vi "To Pretty String (Object).vi"(6 "pretty print? (T)":bool=TRUE, 7 "enable LabVIEW extensions? (T)":bool=TRUE, 8 "error in (no error)":errorcluster, 10 "indent":i32, 11 "JSON Value in":refnum<class "JSON Value.lvclass">) -> (0 "error out":errorcluster, 3 "Pretty Print String":string)   [LabVIEW 2016, in "JSON Value.lvclass"]
doc: "Pretty prints the given JSON data in an easier to read format."
uses:
  JSON Value.lvclass
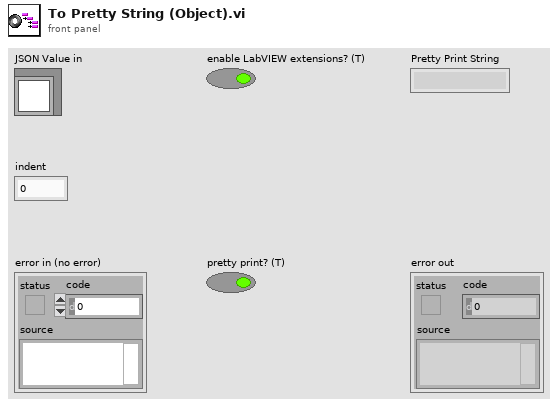
[diagram p1: front panel]
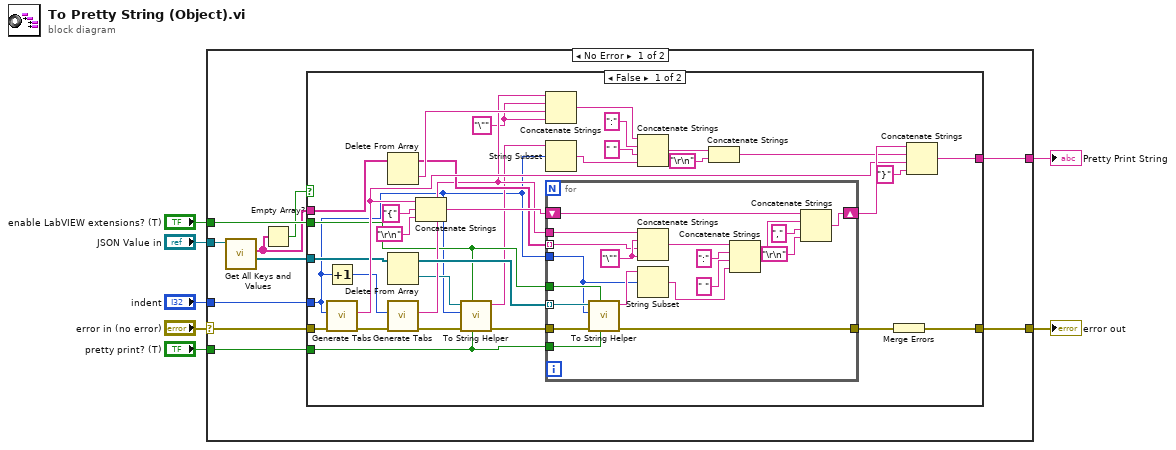
[diagram p0: block diagram]
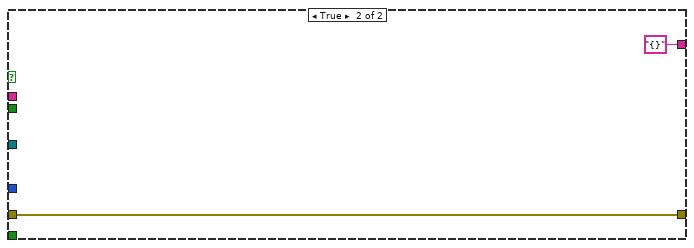
[diagram p2: hidden frame]
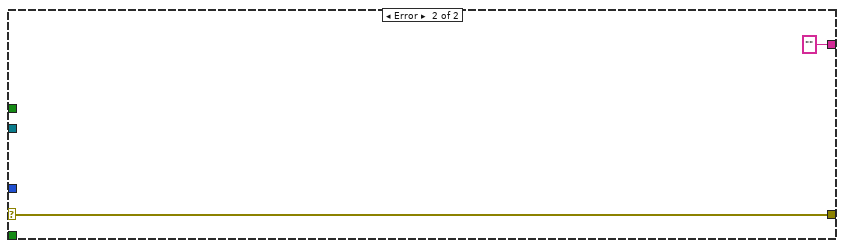
[diagram p3: hidden frame]
diagram:
  n1 = case shown="No Error" "error in (no error)" {
    selector: "error in (no error)" -> [w15 w72]
    tunnel: [w17 ""] -> w7
    tunnel: [w16 w72] -> w6
    tunnel: "JSON Value in" -> [w13 _]
    tunnel: "enable LabVIEW extensions? (T)" -> [w12 _]
    tunnel: "pretty print? (T)" -> [w11 _]
    tunnel: "indent" -> [w8 _]
    frame No Error {
      n2 = call "Get All Keys and Values.vi"("JSON Value in"=w13) -> ("values"=w14:refnum<class "JSON Value.lvclass">[], "keys"=w9:string[])  [unwired: 8 in, 1 out]
      n3 = Empty Array?(array=w9) -> (empty?=w10:bool)
      n4 = case shown="False" w10 {
        tunnel: [w41 "{}"] -> w17
        tunnel: [w48 w70] -> w16
        tunnel: w15 -> [w40 w70]
        tunnel: w14 -> [w39 _]
        tunnel: w12 -> [w31 _]
        tunnel: w11 -> [w30 _]
        tunnel: w9 -> [w29 _]
        tunnel: w8 -> [w18 _]
        frame False {
          w25 = "\"" ("string")
          n5 = Increment(x=w18) -> (x+1=w21:i32)
          n6 = call "Generate Tabs.vi"("error in (no error)"=w40, "indent"=w18) -> ("error out"=w28:errorcluster, "Tabs"=w42:string)  [unwired: 8 in]
          n7 = Delete From Array(array=w29) -> (deleted portion=w38:string, array with subset deleted=w37:string[])  [unwired: 2 in]
          n8 = Delete From Array(array=w39) -> (deleted portion=w34:refnum<class "JSON Value.lvclass">, array with subset deleted=w47:refnum<class "JSON Value.lvclass">[])  [unwired: 2 in]
          n9 = call "Generate Tabs.vi"("error in (no error)"=w28, "indent"=w21) -> ("error out"=w33:errorcluster, "Tabs"=w36:string)  [unwired: 8 in]
          n10 = Concatenate Strings(w42, "{" ("string"), "\r\n") -> (w49:string)
          n11 = call "To String Helper.vi"("pretty print? (T)"=w30, "enable LabVIEW extensions? (T)"=w31, "error in (no error)"=w33, "indent"=w18, "JSON Value in"=w34) -> ("error out"=w32:errorcluster, "String"=w20:string)  [unwired: 5 in]
          n12 = Concatenate Strings(w36, w25, w38, w25) -> (w24:string)
          n13 = String Subset(string=w20, offset (0)=w18) -> (substring=w19:string)  [unwired: 1 in]
          n14 = for {
            tunnel: w47 -> [w57] mode=indexing
            shift-right: [w67] -> w46
            shift-left: w49 -> [w66]
            tunnel: w36 -> [w59]
            tunnel: w37 -> [w62] mode=indexing
            tunnel: w32 -> [w58]
            tunnel: [w56] -> w35
            tunnel: w31 -> [w55]
            tunnel: w30 -> [w54]
            tunnel: w18 -> [w51]
            w64 = "\"" ("string")
            n15 = call "To String Helper.vi"("pretty print? (T)"=w54, "enable LabVIEW extensions? (T)"=w55, "error in (no error)"=w58, "indent"=w51, "JSON Value in"=w57) -> ("error out"=w56:errorcluster, "String"=w53:string)  [unwired: 5 in]
            n16 = Concatenate Strings(w59, w64, w62, w64) -> (w65:string)
            n17 = String Subset(string=w53, offset (0)=w51) -> (substring=w52:string)  [unwired: 1 in]
            n18 = Concatenate Strings(w65, ":" ("string"), " " ("string"), w52) -> (w61:string)
            n19 = Concatenate Strings(w66, w61, "," ("string"), "\r\n") -> (w67:string)
          }
          n20 = Concatenate Strings(w24, ":" ("string"), " " ("string"), w19) -> (w23:string)
          n21 = Concatenate Strings(w23, "\r\n") -> (w45:string)
          n22 = Merge Errors(w35) -> (w48:errorcluster)
          n23 = Concatenate Strings(w46, w45, w42, "}" ("string")) -> (w41:string)
        }
        frame True {
        }
      }
    }
    frame Error {
    }
  }
  "error out" <- w6
  "Pretty Print String" <- w7
